vi "Bind Timestamp (Real).vi"(8 "error in (no error)":errorcluster, 10 "Time Stamp":timestamp, 11 "SQL Statement in":refnum<class "SQL Statement.lvclass">) -> (0 "error out":errorcluster, 3 "SQL Statement out":refnum<class "SQL Statement.lvclass">)   [LabVIEW 2023, in "SQLite.lvlib" / "SQL Statement.lvclass"]
doc: "Bind a LabVIEW Timestampe, converted to DBL, as a SQLite3 Real."
uses:
  SQL Statement.lvclass
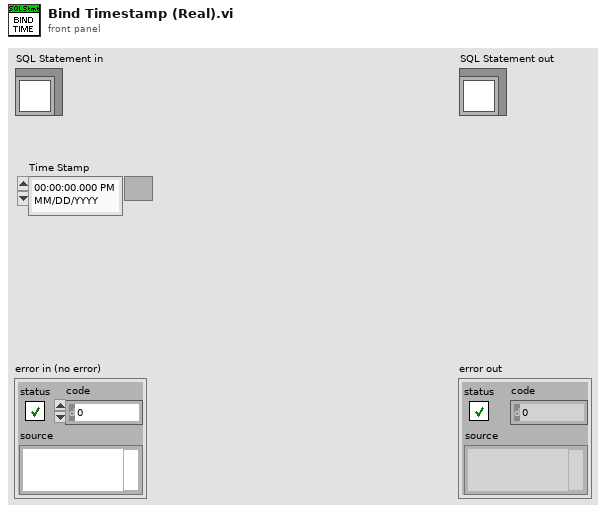
[diagram p1: front panel]
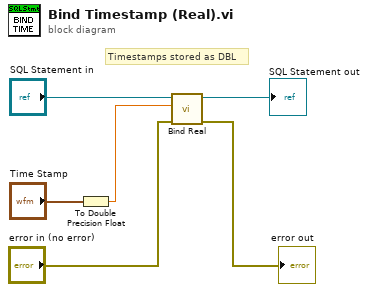
[diagram p0: block diagram]
diagram:
  # "Timestamps stored as DBL"
  n1 = To Double Precision Float(number="Time Stamp") -> (double precision float=w1:dbl)
  n2 = call "Bind Real.vi"("error in (no error)"="error in (no error)", "Real (DBL)"=w1, "SQL Statement in"="SQL Statement in") -> ("error out"=→"error out":errorcluster, "SQL Statement out"=→"SQL Statement out":refnum<class "SQL Statement.lvclass">)  [unwired: 7 in]
